vi "Parse Time String.vi"(4 "Time String":string) -> (6 "Seconds":dbl, 7 "Normalized String":string)   [LabVIEW 2020, in "VolatusGUIElements.lvlib" / "HistorianCharting.lvclass"]
uses:
  HistorianCharting.lvclass
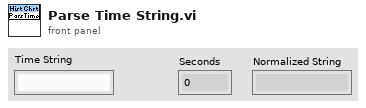
[diagram p1: front panel]
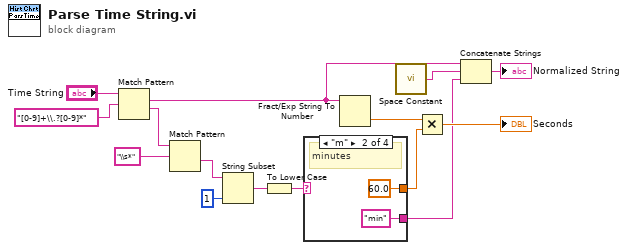
[diagram p0: block diagram]
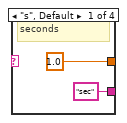
[diagram p2: hidden frame]
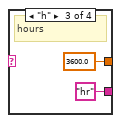
[diagram p3: hidden frame]
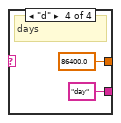
[diagram p4: hidden frame]
diagram:
  n1 = Match Pattern(string="Time String", regular expression="[0-9]+\\.?[0-9]*") -> (match substring=w4:string, after substring=w10:string)  [unwired: 1 in, 2 out]
  n2 = Match Pattern(string=w10, regular expression="\\s*") -> (after substring=w8:string)  [unwired: 1 in, 3 out]
  n3 = String Subset(string=w8, length (rest)=1 ("length (rest)")) -> (substring=w6:string)  [unwired: 1 in]
  n4 = To Lower Case(string=w6) -> (all lower case string=w5:string)
  n5 = case shown="\"m\"" w5 {
    tunnel: [1.0 60.0 3600.0 86400.0] -> w14
    tunnel: ["sec" "min" "hr" "day"] -> w2
    frame "s", Default {
      # "seconds"
    }
    frame "m" {
      # "minutes"
    }
    frame "h" {
      # "hours"
    }
    frame "d" {
      # "days"
    }
  }
  n6 = Fract/Exp String To Number(string=w4) -> (number=w15:dbl)  [unwired: 3 in, 1 out]
  n7 = call <vilib>:"Space Constant.vi"() -> ("String"=w3:string)
  n8 = Multiply(x=w15, y=w14) -> (x*y=→"Seconds":dbl)
  n9 = Concatenate Strings(w4, w3, w2) -> (→"Normalized String":string)
